vi "Locate Subset by Value.vi"(4 "Downsweep?":bool, 7 "Value  Channel":string="B status", 8 "error in":errorcluster, 9 "Start":i64, 10 "threshold y":dbl=139990.0, 11 "File Path":path=path "C:/Data/October_2025/102525/m003_111527_102525.tdms") -> (0 "error out":errorcluster={"status"=TRUE, "code"=-2532, "source"="TDMS Read in loacate subset.vi"}, 1 "Length out":i32, 2 "End Index out":i32=-1, 3 "file path out":path=path "\\\\myhome\\NHMFL/Projects/Pressure/Code/Alex/m006_092123.tdms", 6 "Start Index out":i32=-1)   [LabVIEW 2024]
panel:
  out "fractional index or x":dbl
  in  "group name in":string="p"
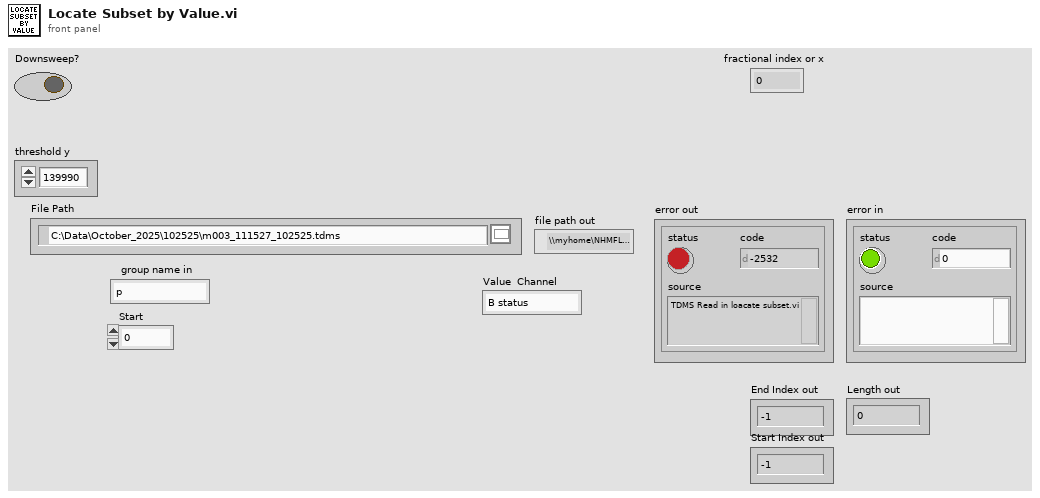
[diagram p1: front panel]
types:
  T1 = enum16{"open", "open or create", "create or replace", "create", "open (read-only)"}
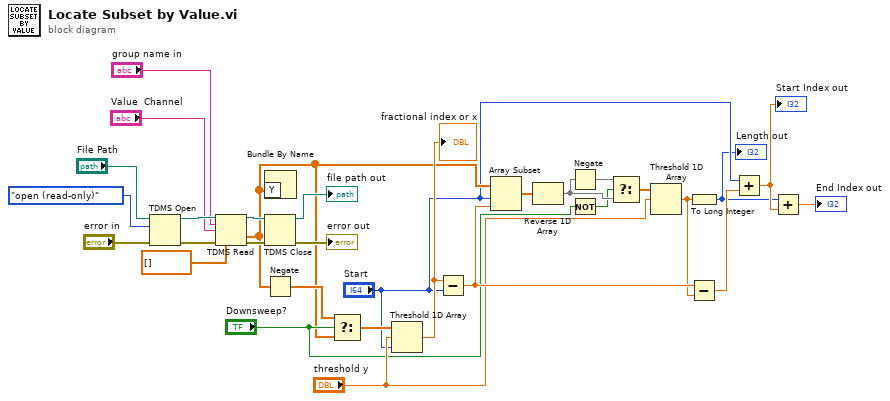
[diagram p0: block diagram]
diagram:
  n1 = TDMS Open(8:"error in", 10:T1."open (read-only)" ("operation (0:open)"), 11:"File Path") -> (0:w28:errorcluster, 3:w29:refnum<k34>)  [unwired: 4 in]
  n2 = TDMS Read(0:w29, 5:"group name in", 7:"Value  Channel", 11:w28, 12:dbl[] []) -> (4:w20:refnum<k34>, 10:w6:dbl[], 15:w21:errorcluster)  [unwired: 3 in, 3 out]
  n3 = Bundle By Name("Y"=w6) -> ()  [unwired: 1 in, 1 out]
  n4 = TDMS Close(8:w21, 11:w20) -> (0:→"error out":errorcluster, 3:→"file path out":path)
  n5 = Negate(x=w6) -> (-x=w9:dbl[])
  n6 = Select(t=w9, s="Downsweep?", f=w6) -> (s? t:f=w8:dbl[])
  n7 = Threshold 1D Array(1:"Start", 2:"threshold y", 3:w8) -> (0:w7:dbl)
  "fractional index or x" <- w7
  n8 = Subtract(x=w7, y="Start") -> (x-y=w17:dbl)
  n9 = Array Subset(array=w6, index="Start", length=w17) -> (w10:dbl[])
  n10 = Reverse 1D Array(array=w10) -> (reversed array=w14:dbl[])
  n11 = Negate(x=w14) -> (-x=w13:dbl[])
  n12 = Not(x="Downsweep?") -> (.not. x?=w12:bool)
  n13 = Select(t=w13, s=w12, f=w14) -> (s? t:f=w15:dbl[])
  n14 = Threshold 1D Array(2:"threshold y", 3:w15) -> (0:w5:dbl)  [unwired: 1 in]
  n15 = To Long Integer(number=w5) -> (32bit integer=w1:i32)
  "Length out" <- w1
  n16 = Subtract(x=w17, y=w5) -> (x-y=w18:dbl)
  n17 = Add(x="Start", y=w18) -> (x+y=w2:dbl)
  "Start Index out" <- w2
  n18 = Add(x=w1, y=w2) -> (x+y=→"End Index out":dbl)
